vi "OutSineAmpGet.vi"(0 "SR865 in":T1, 5 "error in":errorcluster) -> (14 "SR865 out":T1, 16 "Amplitude":dbl caption="Amplitude, V", 19 "error out":errorcluster)   [LabVIEW 2018]
uses:
  SR865.ctl
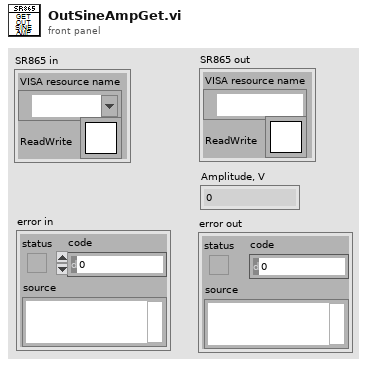
[diagram p1: front panel]
types:
  T1 = typedef "SR865.ctl" = cluster{"VISA resource name":refnum<visa-resource-name>, "ReadWrite":T2}
  T2 = typedef "Semaphore RefNum" = refnum<k1>
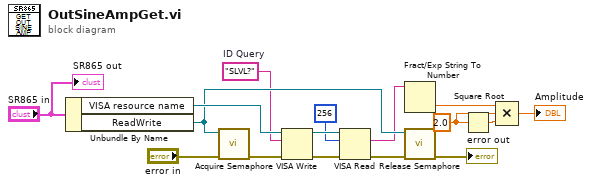
[diagram p0: block diagram]
diagram:
  w3 = 2.0 ("y")
  w5 = "SLVL?"  # ID Query
  n1 = Unbundle By Name("SR865 in") -> ("VISA resource name"=w12:refnum<visa-resource-name>, "ReadWrite"=w7:T2)
  n2 = call <vilib>:"Acquire Semaphore.vi"("error in (no error)"="error in", "semaphore"=w7) -> ("error out"=w11:errorcluster)  [unwired: 3 in, 2 out]
  n3 = VISA Write(VISA resource name=w12, write buffer=w5, error in (no error)=w11) -> (VISA resource name out=w15:refnum<visa-resource-name>, error out=w14:errorcluster)  [unwired: 1 out]
  n4 = VISA Read(VISA resource name=w15, byte count=u32 256, error in (no error)=w14) -> (read buffer=w6:string, error out=w9:errorcluster)  [unwired: 2 out]
  n5 = Fract/Exp String To Number(string=w6) -> (number=w2:dbl)  [unwired: 3 in, 1 out]
  n6 = call <vilib>:"Release Semaphore.vi"("error in (no error)"=w9, "semaphore"=w7) -> ("error out"=→"error out":errorcluster)  [unwired: 4 in, 1 out]
  n7 = Square Root(x=w3) -> (sqrt(x)=w4:dbl)
  n8 = Compound Arithmetic op=MULTIPLY(w2, w3, w4) -> (→"Amplitude":dbl)
  "SR865 out" <- "SR865 in"
